vi "xiC - ZoomImage.vi"(7 "Image Properites":T1, 8 "error in (no error)":errorcluster, 11 "Picture in":refnum<vi>) -> (0 "error out":errorcluster, 3 "Picture out":refnum<vi>)   [LabVIEW 2015]
uses:
  xiCamLib/xiCam/PRM/IMG_FORMAT/IMG_DATA_FORMAT.ctl
  xiCamLib/xiCam/Utils/xiImageManager/xiImageMng - Attributes.ctl
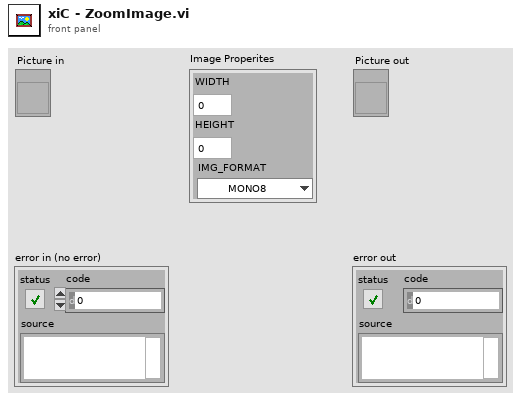
[diagram p1: front panel]
types:
  T1 = typedef "xiImageMng - Attributes.ctl" = cluster{"WIDTH":i32, "HEIGHT":i32, "IMG_FORMAT":T2}
  T2 = typedef "IMG_DATA_FORMAT.ctl" = enum16{"MONO8", "MONO16", "RGB24", "RGB32", "RGBPLANAR", "RAW8", "RAW16"}
  T3 = typedef "LVBoundsTypeDef.ctl" = cluster{"Width":u32, "Height":u32}
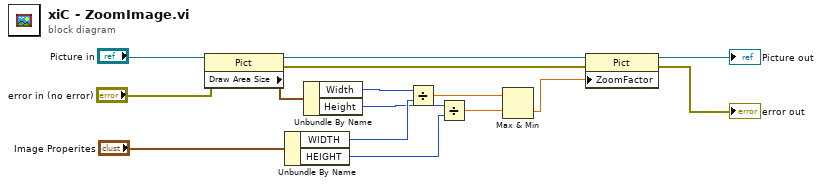
[diagram p0: block diagram]
diagram:
  n1 = property class="Pict"(reference="Picture in", error in="error in (no error)") -> (reference out=w14:refnum<vi>, error out=w2:errorcluster, "Draw Area Size"=w15:T3)
  n2 = Unbundle By Name("Image Properites") -> ("WIDTH"=w10:i32, "HEIGHT"=w8:i32)
  n3 = Unbundle By Name(w15) -> ("Width"=w12:u32, "Height"=w9:u32)
  n4 = Divide(x=w12, y=w10) -> (x/y=w7:dbl)
  n5 = Divide(x=w9, y=w8) -> (x/y=w6:dbl)
  n6 = Max & Min(x=w7, y=w6) -> (min(x,y)=w4:dbl)  [unwired: 1 out]
  n7 = property class="Pict"(reference=w14, error in=w2, "ZoomFactor"=w4) -> (reference out=→"Picture out":refnum<vi>, error out=→"error out":errorcluster)
